vi "__Update Cloud List.vi"(8 "error in (no error)":errorcluster, 9 "Bucket":string, 10 "Path to list":string, 11 "FileManager Ctl Refs in":T1) -> (0 "error out":errorcluster, 3 "FileManager Ctl Refs out":T1)   [LabVIEW 2011]
doc: "Queries the objects that reside in the selected bucket under the specified path and updates the Cloud list with the items."
uses:
  __File manager Data type.ctl
  <vilib>/Utility/miscctls.llb/LVRowAndColumnUnsignedTypeDef.ctl
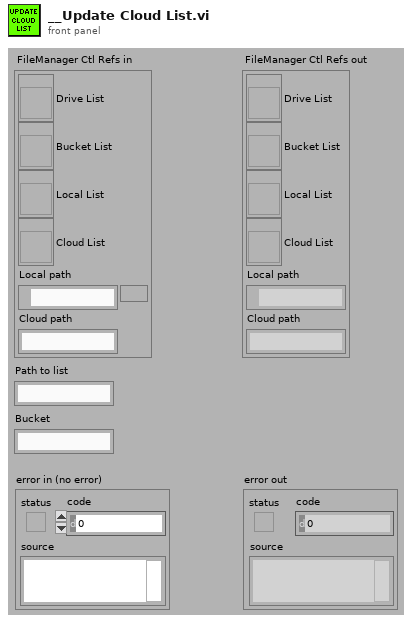
[diagram p1: front panel]
types:
  T1 = typedef "__File manager Data type.ctl" = cluster{"Drive List":refnum<vi>, "Bucket List":refnum<vi>, "Local List":refnum<vi>, "Cloud List":refnum<vi>, "Local path":path, "Cloud path":string}
  T2 = typedef "__Cloud Object Info type.ctl" = cluster{"Name":string, "Size (bytes)":u64, "Last modified":timestamp, "Storage Class":T3}
  T3 = typedef "LV Interface for Amazon S3.lvlib/AMZ_S3_Storage Class.ctl" = enum16{"STANDARD", "REDUCED_REDUNDANCY"}
  T4 = typedef "LVRowAndColumnUnsignedTypeDef.ctl" = cluster{"Row":u32, "Column":u32}
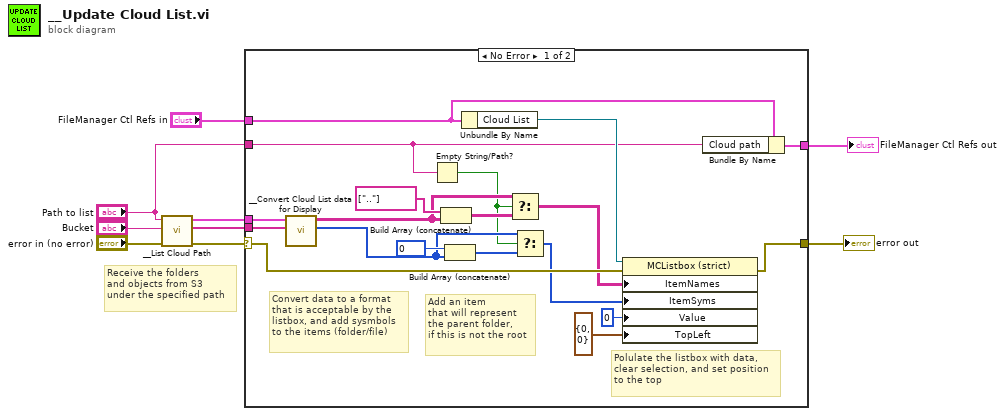
[diagram p0: block diagram]
diagram:
  # "Receive the folders\nand objects from S3\nunder the specified path"
  n1 = call "__List Cloud Path.vi"("error in (no error)"="error in (no error)", "Bucket"="Bucket", "Path"="Path to list") -> ("error out"=w4:errorcluster, "Folders"=w2:string[], "Objects"=w3:T2[])  [unwired: 6 in]
  n2 = case shown="No Error" w4 {
    selector: w4 -> [w22 w29]
    tunnel: [w28 w29] -> w9
    tunnel: "FileManager Ctl Refs in" -> [w27 w30]
    tunnel: [w26 w30] -> w7
    tunnel: w3 -> [w23 _]
    tunnel: w2 -> [w24 _]
    tunnel: "Path to list" -> [w13 _]
    frame No Error {
      # "Add an item\nthat will represent\nthe parent folder,\nif this is not the root"
      # "Convert data to a format\nthat is acceptable by the\nlistbox, and add sysmbols\nto the items (folder/file)"
      # "Polulate the listbox with data,\nclear selection, and set position\nto the top"
      n3 = call "__Convert Cloud List data for Display.vi"("Folders"=w24, "Objects"=w23) -> ("Symbols"=w15:i32[], "List data"=w17:string[][])  [unwired: 8 in]
      n4 = Empty String/Path?(string/path=w13) -> (empty?=w12:bool)
      n5 = Build Array (concatenate)(string[] [".."], w17) -> (w19:string[][])
      n6 = Build Array (concatenate)(0, w15) -> (w18:i32[])
      n7 = Unbundle By Name(w27) -> ("Cloud List"=w25:refnum<vi>)
      n8 = Select(t=w17, s=w12, f=w19) -> (s? t:f=w16:string[][])
      n9 = Select(t=w15, s=w12, f=w18) -> (s? t:f=w14:i32[])
      n10 = property class="MCListbox (strict)"(reference=w25, error in=w22, "ItemNames"=w16, "ItemSyms"=w14, "Value"=0, "TopLeft"=T4 {"Row"=0, "Column"=0} ("Top Left Visible Cell")) -> (error out=w28:errorcluster)  [unwired: 1 out]
      n11 = Bundle By Name(cluster=w27, "Cloud path"=w13) -> (w26:T1)
    }
    frame Error {
    }
  }
  "FileManager Ctl Refs out" <- w7
  "error out" <- w9
